vi "Increment Error Count.vi"(8 "error in (no error)":errorcluster, 11 "Result Table.lvclass":refnum<class "Result Table V2.lvclass">) -> (0 "error out":errorcluster, 3 "Result Table":refnum<class "Result Table V2.lvclass">)   [LabVIEW 2020, in "Result Table V2.lvclass"]
uses:
  Result Table V2.lvclass
  Result Table V2.lvclass/Result Table V2.ctl
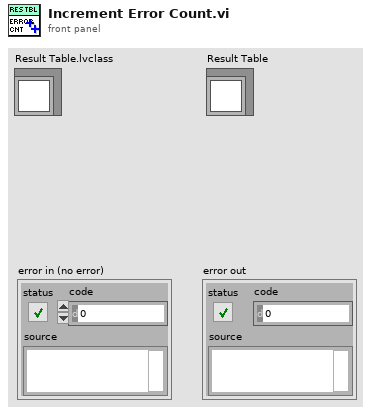
[diagram p1: front panel]
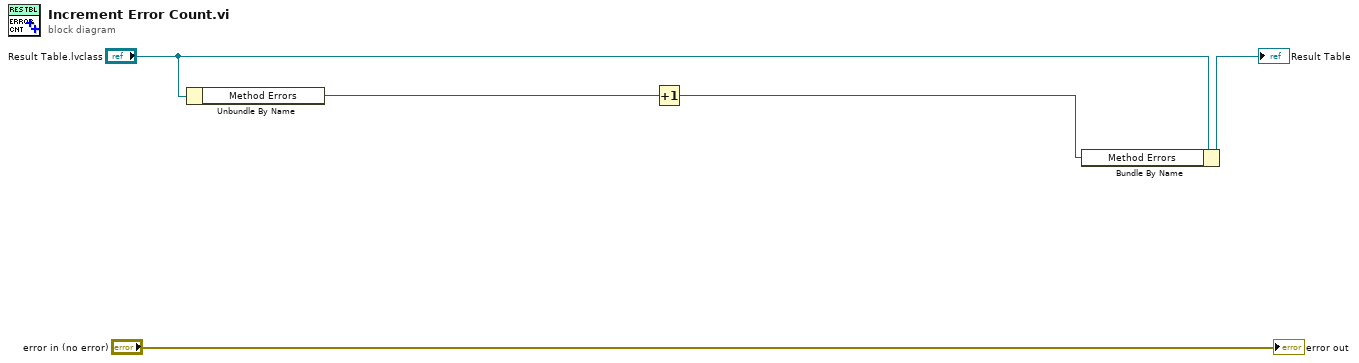
[diagram p0: block diagram]
diagram:
  n1 = Unbundle By Name("Result Table.lvclass") -> ("Method Errors"=w2:u32)
  n2 = Increment(x=w2) -> (x+1=w1:u32)
  n3 = Bundle By Name(cluster="Result Table.lvclass", "Method Errors"=w1) -> (→"Result Table":refnum<class "Result Table V2.lvclass">)
  "error out" <- "error in (no error)"
